vi "fpga.complete.test.harness.vi"() -> ()   [LabVIEW 2020]
uses:
  <vilib>/Platform/TimedLoop/XDataNode/XDataNode.xnode
  <vilib>/Platform/TimedLoop/XDataNode/nitl_modes.ctl
  <vilib>/Platform/TimedLoop/XDataNode/XDNodeRunTimeDep.lvlib
  <vilib>/Platform/TimedLoop/XDataNode/wakeup.ctl
  <vilib>/Platform/TimedLoop/XDataNode/timing_clust.ctl
  <vilib>/rvi/LocalResourceManager/LocalResourceManager.xnode
  <vilib>/rvi/DataTransferAndStorage/Container/XNode/niFpgaContainer.xnode
  <vilib>/rvi/FIFO/Fifo_Resource/niFpgaFifoEmulationRefIn.vi
  <vilib>/rvi/DataTransferAndStorage/Container/Common/niFpgaContainerGetUniqueNameForEmu.vi
  <vilib>/rvi/DataTransferAndStorage/Container/Common/niFpgaContainerSetEmuInfo.vi
  <vilib>/rvi/eio/common/nirviEmuReportErrorAndStop.vi
  <vilib>/rvi/interface/RandomDataEmulation/nirviRandomDataFpgaReadWriteTemplate.vi
  Test/test.data.in.ctl
  <vilib>/rvi/interface/RandomDataEmulation/nirviRandomDataFpgaMultiElementTemplate.vi
  <instrlib>/_niInstr/Network/Types/v1/IPv4 Address.ctl
  <instrlib>/_niInstr/Network/Types/v1/niInstr Network Types v1.lvlib
  <instrlib>/_niInstr/Network/Types/v1/MAC Address.ctl
panel:
  in  "MAC Address":T1=[220, 166, 50, 109, 145, 21] format="%.0x"
  in  "Dest Port":u16=6001
  in  "IP Address":T2=[192, 168, 1, 60]
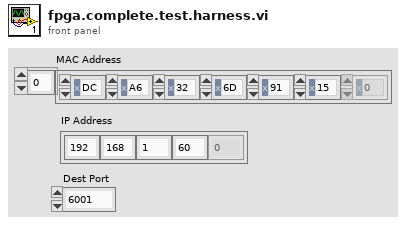
[diagram p1: front panel]
types:
  T1 = typedef "niInstr Network Types v1.lvlib/MAC Address.ctl" = u8[]
  T2 = typedef "niInstr Network Types v1.lvlib/IPv4 Address.ctl" = u8[]
  T3 = typedef "XDNodeRunTimeDep.lvlib/timing_clust.ctl" = cluster{"Expected End [f-1]":u64, "Actual End [f-1]":u64, "Finished Late? [f-1]":bool, "Expected End [i-1]":u64, "Actual End [i-1]":u64, "Finished Late? [i-1]":bool, "Expected Start [i]":u64, "Actual Start [i]":u64, "Expected Start [f]":u64, "Actual Start [f]":u64, "Source Name":string, "Structure Name":string, "Period":i64, "Deadline":i64, "Offset":i64, "Start":i64, "Priority":i32, "Timeout":i32, "Mode":T4, "Wakeup Reason":T5, "Error":errorcluster, "Source Type":string, "Secondary Source Type":string, "Global End Time":u64, "Global Start Time":u64, "Frame Duration":u64, "Iteration Duration":u64, "Assigned CPU":i32, "I/O Scan Engine Mode":u32}
  T4 = typedef "XDNodeRunTimeDep.lvlib/nitl_modes.ctl" = enum32{"No Change", "Process missed periods, maintain original phase", "Discard missed periods, maintain original phase", "Process missed periods, ignore original phase", "Discard missed periods, ignore original phase"}
  T5 = typedef "XDNodeRunTimeDep.lvlib/wakeup.ctl" = enum32{"Normal", "Aborted", "Asynchronous wakeup", "Timing source error", "Timed loop error", "Timeout"}
  T6 = typedef "test.data.in.ctl" = cluster{"data":u8, "end_of_frame":bool}
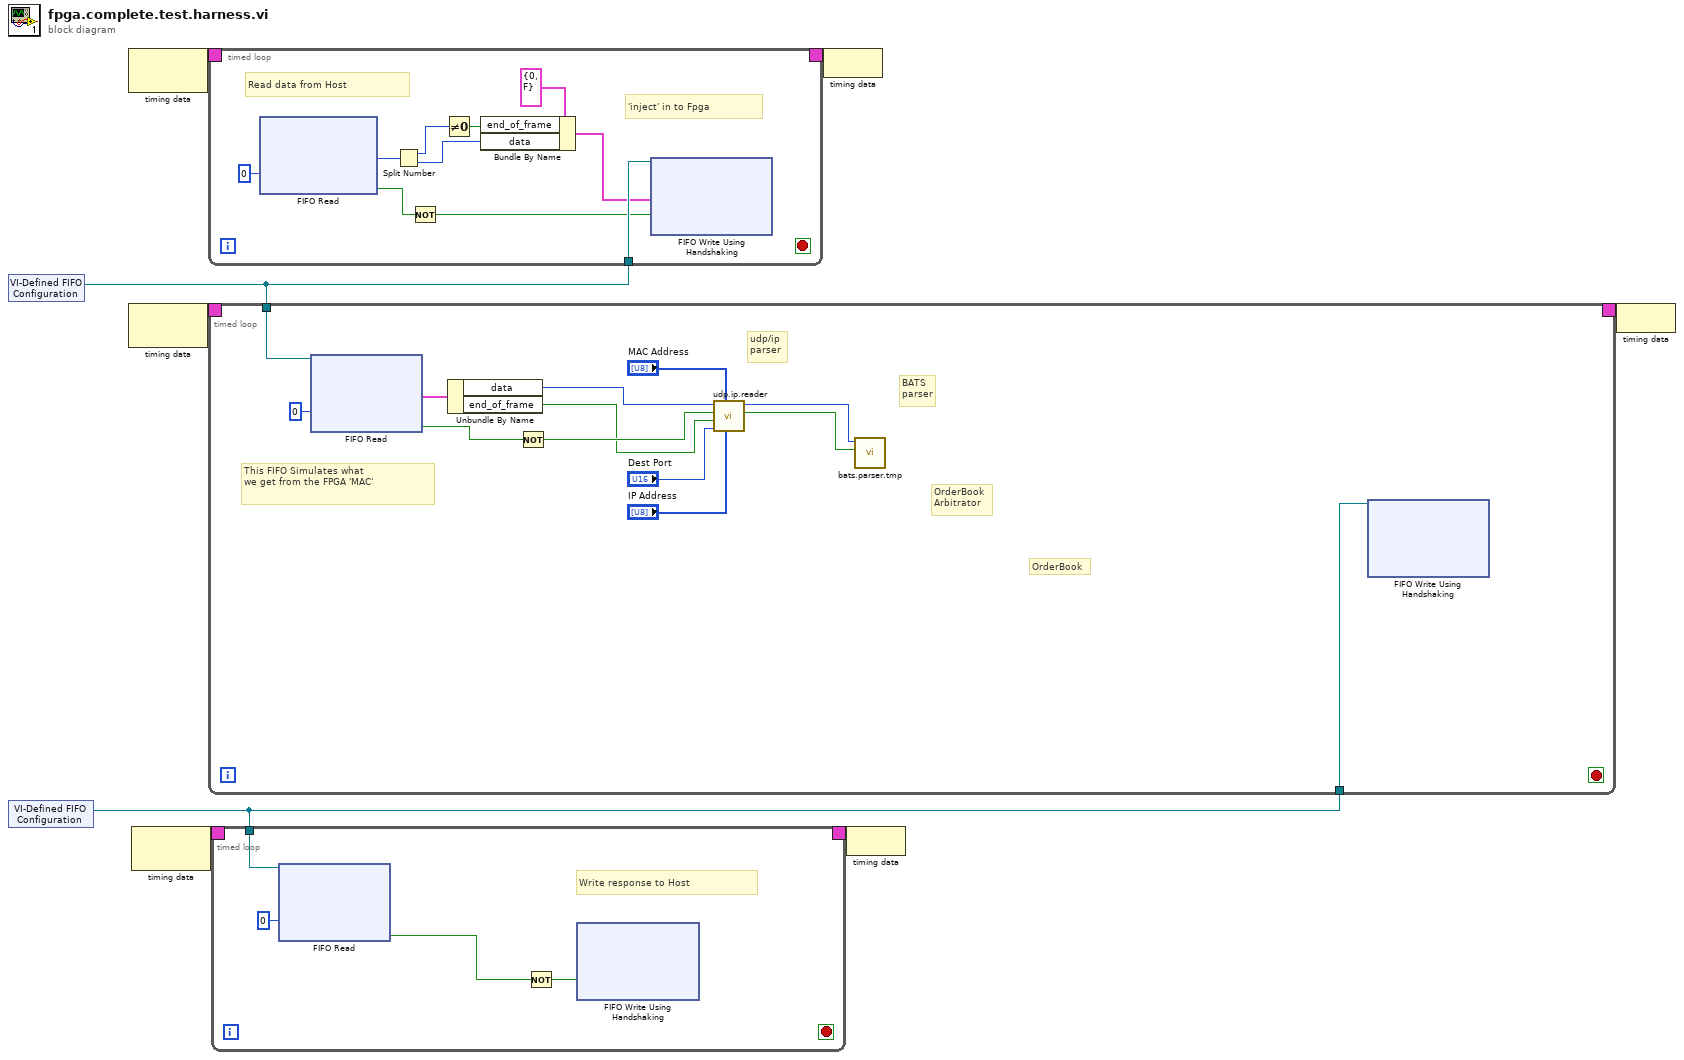
[diagram p0: block diagram]
diagram:
  n1 = xnode "VI-Defined FIFO Configuration"() -> ("FIFO Out"=w4:refnum<k21>)
  n2 = xnode "VI-Defined FIFO Configuration"() -> ("FIFO Out"=w1:refnum<k21>)
  n3 = node-c288() -> (w8:T3)  [unwired: 1 in]
  n4 = node-c288() -> (w6:T3)  [unwired: 1 in]
  n5 = node-c288() -> (w3:T3)  [unwired: 1 in]
  n6 = timed-loop {
    timing: w8 -> [_]
    timing-out: [_] -> w7
    tunnel: w4 -> [w18]
    stop <- _ stop-if-true
    # "'inject' in to Fpga"
    # "Read data from Host"
    n7 = xnode "FIFO Read"("Timeout"=0) -> ("Element"=w14:u16, "Timed Out?"=w16:bool)  [unwired: 1 in, 1 out]
    n8 = Split Number(x=w14) -> (hi(x)=w10:u8, lo(x)=w12:u8)
    n9 = Not(x=w16) -> (.not. x?=w15:bool)
    n10 = Not Equal To 0?(x=w10) -> (x != 0?=w11:bool)
    n11 = Bundle By Name(cluster=T6 {"data"=0, "end_of_frame"=FALSE} ("Cluster"), "end_of_frame"=w11, "data"=w12) -> (w9:T6)
    n12 = xnode "FIFO Write Using Handshaking"("Element"=w9, "Input Valid"=w15, "FIFO In"=w18) -> ()  [unwired: 2 out]
  }
  n13 = timed-loop {
    timing: w6 -> [_]
    timing-out: [_] -> w5
    tunnel: w4 -> [w33]
    tunnel: w1 -> [w29]
    stop <- _ stop-if-true
    # "OrderBook\nArbitrator"
    # "BATS\nparser"
    # "udp/ip\nparser"
    # "OrderBook"
    # "This FIFO Simulates what\nwe get from the FPGA 'MAC'"
    n14 = xnode "FIFO Read"("Timeout"=0, "FIFO In"=w33) -> ("Element"=w31:cluster{"data":u8, "end_of_frame":bool}, "Timed Out?"=w30:bool)  [unwired: 1 out]
    n15 = Unbundle By Name(w31) -> ("data"=w25:u8, "end_of_frame"=w23:bool)
    n16 = Not(x=w30) -> (.not. x?=w24:bool)
    n17 = call "udp.ip.reader.vi"("IP Address"="IP Address", "MAC Address"="MAC Address", "Dest Port"="Dest Port", "end_of_frame"=w23, "data_valid"=w24, "data"=w25) -> ("udp_data valid_out"=w21:bool, "udp_data_out"=w22:u8)  [unwired: 3 in, 1 out]
    n18 = call "bats.parser.tmp.vi"("data_valid"=w21, "data"=w22) -> ()  [unwired: 9 in, 1 out]
    n19 = xnode "FIFO Write Using Handshaking"("FIFO In"=w29) -> ()  [unwired: 2 in, 2 out]
  }
  n20 = timed-loop {
    timing: w3 -> [_]
    timing-out: [_] -> w2
    tunnel: w1 -> [w39]
    stop <- _ stop-if-true
    # "Write response to Host"
    n21 = xnode "FIFO Read"("Timeout"=0, "FIFO In"=w39) -> ("Timed Out?"=w37:bool)  [unwired: 2 out]
    n22 = Not(x=w37) -> (.not. x?=w36:bool)
    n23 = xnode "FIFO Write Using Handshaking"("Input Valid"=w36) -> ()  [unwired: 2 in, 2 out]
  }
  n24 = node-c288(w7) -> ()
  n25 = node-c288(w2) -> ()
  n26 = node-c288(w5) -> ()
